vi "Enter Idle Mode [STX].vi"(7 "Micropulse # In":i32, 8 "error in (no error)":errorcluster, 9 "Erase All? (def T)":bool) -> (0 "error out":errorcluster, 5 "Micropulse # Out":i32)   [LabVIEW 2026, in "MicroPulse_Driver.lvlib"]
doc: "To enter idle mode with no test displayed.\n\nThis command is useful for suspending pulser activity.\n\nParameters:\n[option] :\n If omitted all test activity is stopped and any remaining test data is sent to the host.\n\nIf=1 All test activity is stopped, the contents of the data buffer are erased, and a message is sent to indicate completion. For the format of the output message see the MicroPulse Output Messages section. Prior to the STX 1 complete message, MicroPulse may also send a series of header 0 messages (single byte). This is to ensure that the last data set has been completed prior to the STX 1 complete message. This maintains message synchronisation with the host. Header 0 messages should be discarded."
uses:
  MicroPulse_Driver.lvlib
  <instrlib>/MicroPulse/Public/Data/Datatypes/MP - instrument type.ctl
  Private/MP-Registry Action-Enum.ctl
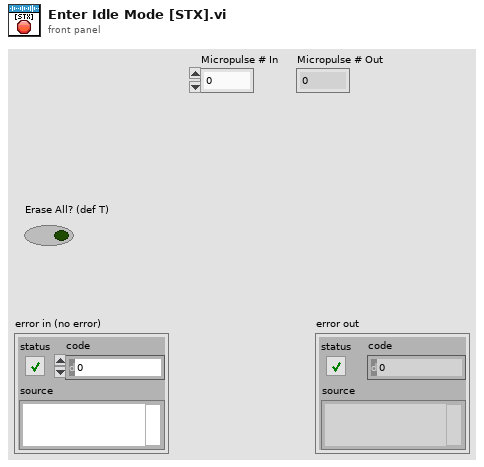
[diagram p1: front panel]
types:
  T1 = typedef "MicroPulse_Driver.lvlib/MP - instrument type.ctl" = enum16{"MicroPulse 5", "LT1", "LT2", "LTPA", "MPLT", "MicroPulse 6", "PipeScanner", "<MicroPulse>", "Micropulse 4", "Simulated Data"}
  T2 = typedef "MicroPulse_Driver.lvlib/MP-Registry Data-Cluster.ctl" = cluster{"Instrument Type":T1, "Serial #":u64, "Sample Frequency":T3, "dt (us)":dbl, "DOF":T4, "Material Velocity":dbl, "Asynch Reads":T5, "NUM of Tests":u32, "System Details":T6, "Gates":T8[], "Encoders":T15[], "CMD LUT":variant, "Command List":string}
  T3 = typedef "MicroPulse_Driver.lvlib/MP - sample frequency.ctl" = enum16{"Use Default", "200MHz (LT2 only)", "100MHz", "50MHz", "25MHz", "10MHz"}
  T4 = typedef "MicroPulse_Driver.lvlib/MP - data output format.ctl" = enum16{"", "8-bit Mode", "10-bit Mode", "12-bit Mode", "16-bit Mode", "8-bit Log Mode", "12-bit Packed Mode"}
  T5 = typedef "MicroPulse_Driver.lvlib/MP - asynch read mode.ctl" = enum16{"Disabled", "Enabled"}
  T6 = typedef "MicroPulse_Driver.lvlib/MP - general system status.ctl" = cluster{"System Type":T1, "Serial No.":u64, "Channels":cluster{"Conv":u8, "PA":u16, "Extra":u32}, "Sample Frequency":cluster{"Default":u8, "Actual":u8}, "Software Versions":string, "Data Output Format":cluster{"Default":T4, "Actual":T4}, "Temperatures":cluster{"System":u8, "Processor":u8, "Slave Sys":u8, "Slave Proc":u8}, "Tx Buffer Size":u32, "System Error":string, "No. of Cards":u8, "DAC Gain":i16, "Uptimes":cluster{"since Power":u32, "since RSTS":u32, "since SRST":u32}, "Voltages":cluster{"Nominal":dbl, "Measured":dbl, "Difference":dbl}[], "Interface Cards":T7[]}
  T7 = typedef "MicroPulse_Driver.lvlib/MP - interface card status.ctl" = cluster{"Status":u8, "Map":u8, "Board - T":u8, "FPGA - T":u8, "PAIF Status":string, "Version":string}
  T8 = typedef "MicroPulse_Driver.lvlib/MP - Registry Gates.ctl" = cluster{"Display Gate":T9, "ETM Mode":T10, "Echo Gate":T11, "Insp Gates":T12[]}
  T9 = typedef "MicroPulse_Driver.lvlib/MP - display gate.ctl" = cluster{"Start":dbl, "Length":dbl}
  T10 = typedef "MicroPulse_Driver.lvlib/MP - echo gate mode.ctl" = enum16{"Echo Trigger OFF", "Echo Gate Display Mode", "Echo Trigger ON", "Multi Gate or FMC Mode", "Reserved", "PA - Echo Trigger ON"}
  T11 = typedef "MicroPulse_Driver.lvlib/MP - echo gate parameters.ctl" = cluster{"Start (us)":dbl, "Length (us)":dbl, "Threshold":u16, "Colour":u32}
  T12 = typedef "MicroPulse_Driver.lvlib/MP - multigate inspection gate parameters.ctl" = cluster{"Start (us)":dbl, "Length (us)":dbl, "Threshold":u16, "Enabled?":bool, "Max # Peaks":u16, "Hysteresis":T13, "Mode":T14, "Inverted?":bool, "Colour ":u32}
  T13 = typedef "MicroPulse_Driver.lvlib/MP - hysteresis level.ctl" = enum16{"None", "3dB", "6dB", "9dB", "12dB"}
  T14 = typedef "MicroPulse_Driver.lvlib/MP - multigate mode.ctl" = enum16{"1st Peak in Gate", "Largest Peak In Gate", "All Peaks In Gate", "1st Threshold Crossing"}
  T15 = typedef "MicroPulse_Driver.lvlib/MP - encoder settings.ctl" = cluster{"Encoder Type":T16, "Counts/mm":u32, "Enable Termination?":bool, "Multiplier":u32, "Backlash Period (s)":dbl, "Encoder Filter":u32}
  T16 = typedef "MicroPulse_Driver.lvlib/MP - encoder type.ctl" = enum16{"Quadrature", "Step/Direction"}
  T17 = typedef "MicroPulse_Driver.lvlib/TCP config.ctl" = cluster{"Connection ID":refnum<k5>, "IP address":string, "host port":u16, "OC timeout":i32, "Read timeout":i32, "Write timeout":i32}
  T18 = typedef "MicroPulse_Driver.lvlib/MP-Registry Action-Enum.ctl" = enum16{"Read", "Add Test", "Add Command", "Add Gate Command", "Add Encoder Command", "Clear Command  List", "Set Registry", "Set System Details", "Set DOF", "Set Velocity", "Disable Asynch Reads", "Enable Asynch Reads", "Add Connection", "Disconnect", "Shutdown"}
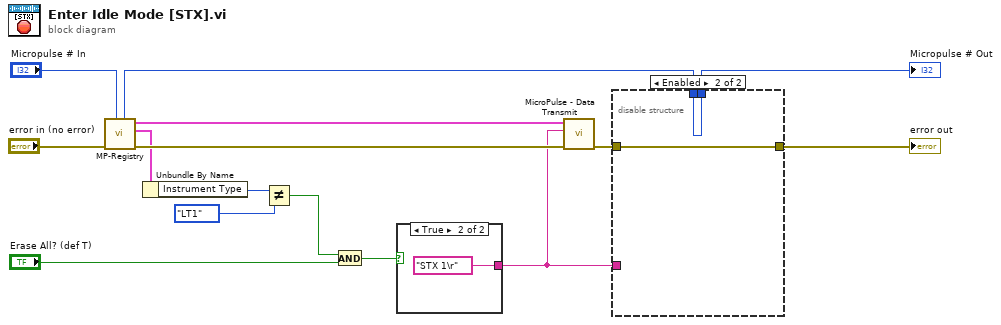
[diagram p0: block diagram]
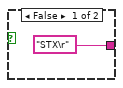
[diagram p2: hidden frame]
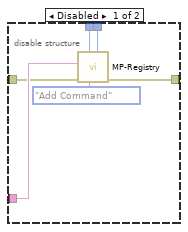
[diagram p3: hidden frame]
diagram:
  n1 = call "MP-Registry.vi"("Micropulse # In"="Micropulse # In", "error in (no error)"="error in (no error)") -> ("error out"=w13:errorcluster, "Micropulse Data"=w4:T2, "TCP config"=w12:T17, "Micropulse # Out"=w9:i32)  [unwired: 6 in]
  n2 = Unbundle By Name(w4) -> ("Instrument Type"=w3:T1)
  n3 = Not Equal?(x=w3, y=MP_-_instrument_type."LT1") -> (x != y?=w1:bool)
  n4 = And(x=w1, y="Erase All? (def T)") -> (x .and. y?=w5:bool)
  n5 = case shown="True" w5 {
    tunnel: ["STX\r" ("format string") "STX 1\r" ("format string")] -> w7
    frame False {
    }
    frame True {
    }
  }
  n6 = call "MicroPulse - Data Transmit.vi"("error in (no error)"=w13, "data"=w7, "TCP config"=w12) -> ("error out"=w11:errorcluster)  [unwired: 6 in, 2 out]
  n7 = disable-structure shown="Enabled" {
    disable-tunnel: w7 -> [w23 _]
    disable-tunnel: w11 -> [w21 w24]
    disable-tunnel: [w20 w24] -> w10
    disable-tunnel: w9 -> [w19 w25]
    disable-tunnel: [w18 w25] -> w8
    frame Disabled {
      n8 = call "MP-Registry.vi"("Action"=MP-Registry_Action-Enum."Add Command", "Micropulse # In"=w19, "error in (no error)"=w21, "Data in"=w23) -> ("error out"=w20:errorcluster, "Micropulse # Out"=w18:i32)  [unwired: 4 in, 2 out]
    }
    frame Enabled {
    }
  }
  "error out" <- w10
  "Micropulse # Out" <- w8
